vi "LJstreamM exec SignedMSWLSW.vi"(8 "error in (no error)":errorcluster, 10 "LSB":u32, 11 "MSB":u32) -> (0 "error out":errorcluster, 3 "(MSB << 16 ) | LSB":u32)   [LabVIEW 2025]
doc: "Similar to the Formula Node function, but with variables that can be entered on the front panel."
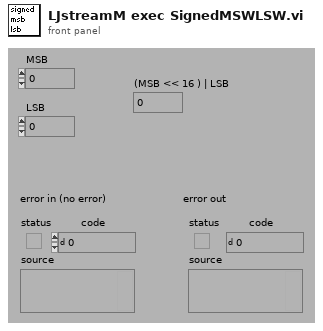
[diagram p1: front panel]
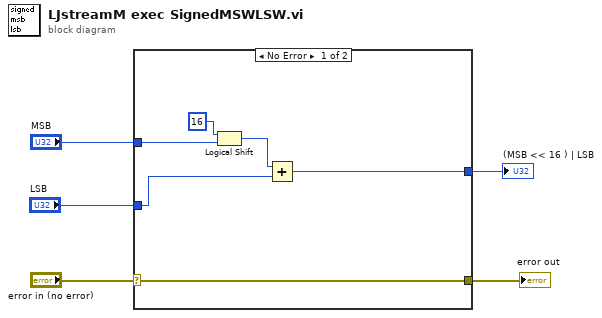
[diagram p0: block diagram]
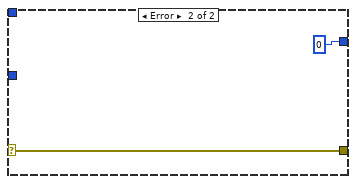
[diagram p2: hidden frame]
diagram:
  n1 = case shown="No Error" "error in (no error)" {
    selector: "error in (no error)" -> [w8 w13]
    tunnel: [w8 w13] -> w5
    tunnel: "MSB" -> [w7 _]
    tunnel: [w9 0] -> w3
    tunnel: "LSB" -> [w10 _]
    frame No Error {
      n2 = Logical Shift(y=u32 16 ("x"), x=w7) -> (x << y=w11:u32)
      n3 = Add(x=w11, y=w10) -> (x+y=w9:u32)
    }
    frame Error {
    }
  }
  "error out" <- w5
  "(MSB << 16 ) | LSB" <- w3
